vi "CVFinder.vi"() -> ()   [LabVIEW 2017]
uses:
  <vilib>/Utility/file.llb/Write Delimited Spreadsheet (string).vi
  <vilib>/Utility/file.llb/Write Delimited Spreadsheet (DBL).vi
  <instrlib>/Agilent E4980/Agilent E4980.lvlib
  <vilib>/Analysis/NI_AALPro.lvlib
panel:
  in  "Save data after run":bool=TRUE
  in  "Save NW Image to:":path=path "C:/Users/Noah/Desktop/NW_test.png" caption="Save CV Data to:"
  in  "stoploop":bool
  out "Steps":dbl
  out "Width (mm)":dbl
  out "Capacitance (pF)":dbl
  out "NW":cluster{dbl[], ext[unit][]}(graph) caption="Primary"
  out "1_C2V":cluster{dbl[], dbl[]}(graph)={[-1.0], [1.8568866883502444e+20]} caption="Primary"
  in  "Save CV Data to:":path=path "C:/Users/Noah/Desktop/CV_test.txt"
  out "CV":cluster{dbl[], dbl[]}(graph)={[-1.0], [73.385]} caption="Primary"
  in  "Manual Impedance Range (3: 100 Ohms) 2":i32(ring)=3 items=["100m", "1", "10", "100", "300", "1K", "3K", "10K", "30K", "100K"]
  in  "Relative Permittivity, er":dbl=11.68 caption="Permittivity (pF/cm)"
  in  "Signal Frequency (kHz)":dbl=1000.0
  in  "Voltage Increment (V)":dbl=0.05
  in  "Final Voltage (V)":dbl=3.0
  in  "Initial Voltage (V)":dbl=0.1
  in  "Area (cm^2)":dbl=0.005153 format="%#_6e"
  in  "Enable Auto Range (T:Enable) 2":bool=TRUE
  in  "Signal Type (0: Voltage) 2":u16(ring) items=["Voltage"]
  in  "Function (0: Cp-D) 2":u16(ring)=1 items=["Cp-D", "Cp-Q", "Cp-G", "Cp-Rp", "Cs-D", "Cs-Q", "Cs-Rs", "Lp-D", "Lp-Q", "Lp-G", "Lp-Rp", "Lp-Rdc", "Ls-D", "Ls-Q", "Ls-Rs", "Ls-Rdc", "R-X", "Z-thd", "Z-thr", "G-B", "Y-thd", "Y-thr", "Vdc-Idc"]
  in  "error in (no error)":errorcluster
  in  "VISA resource name":refnum<visa-resource-name>="USB0::0x0957::0x0909::MY46101893::INSTR"
  out "Q":dbl
  # "e0 = 0.088542 pF/cm"
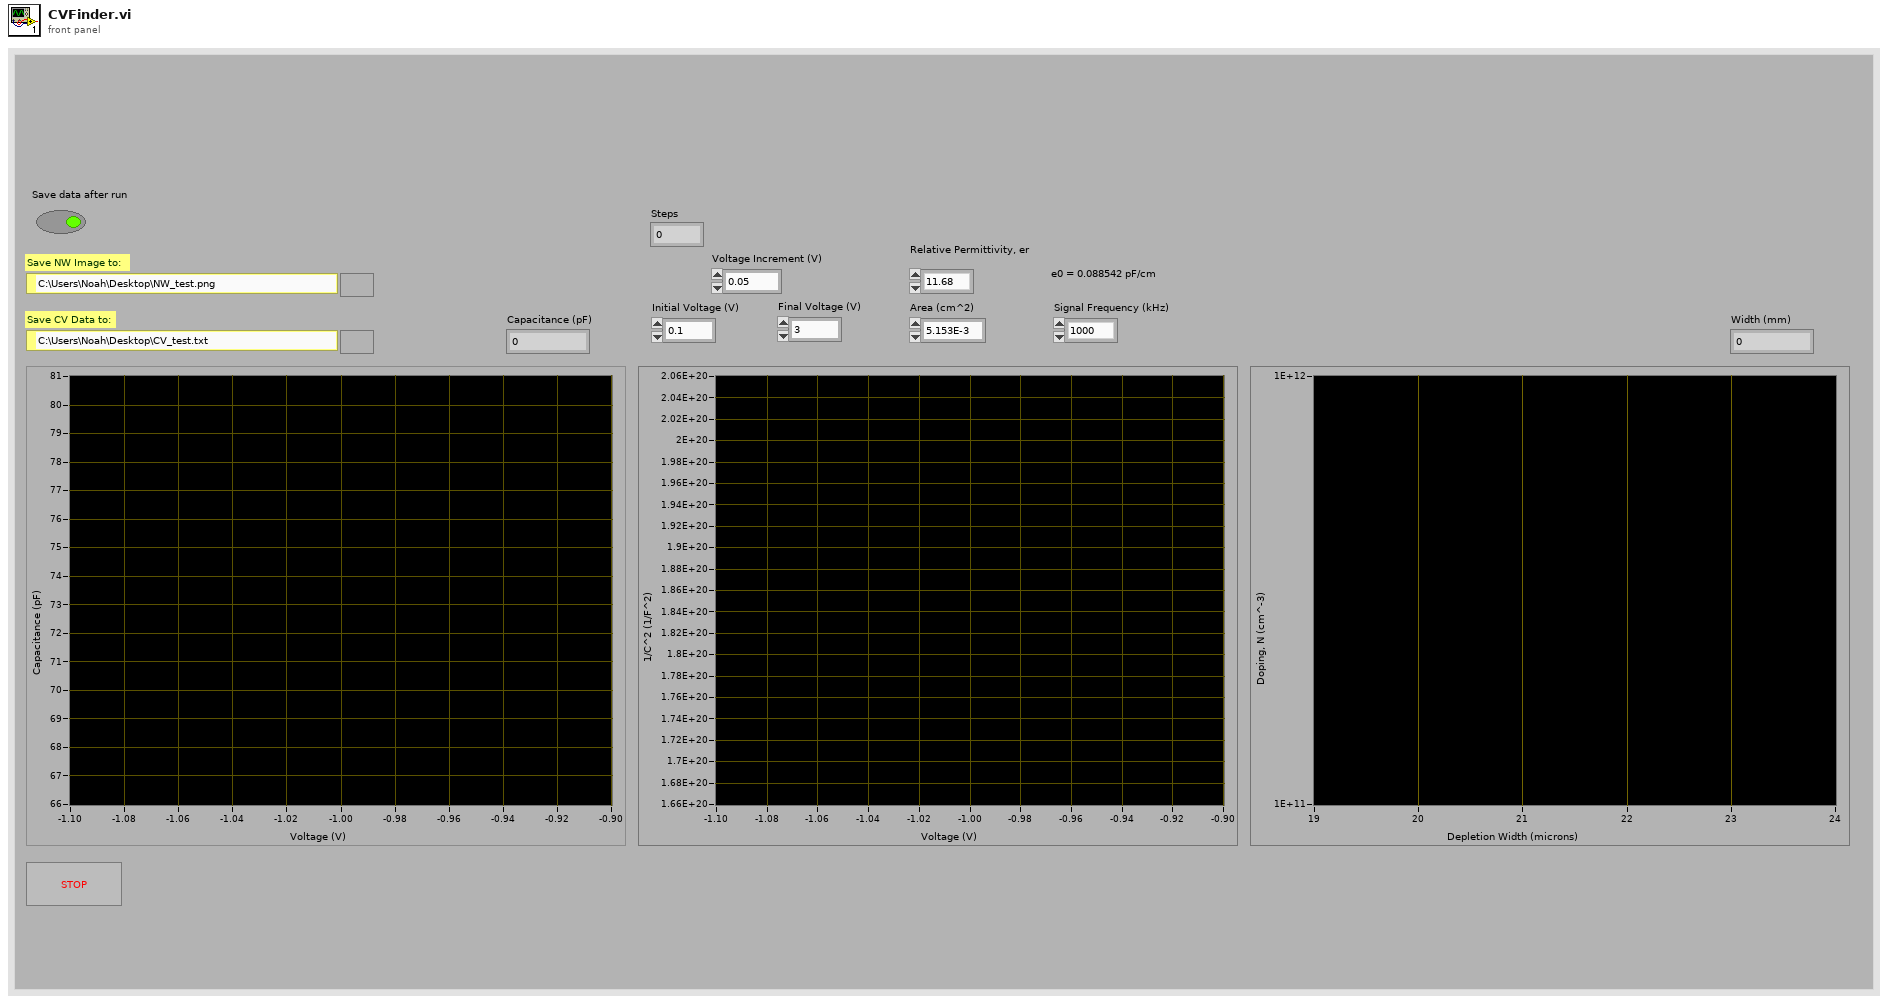
[diagram p1: front panel]
types:
  T1 = typedef "imagedata.ctl" = cluster{"image type":i32, "image depth":i32, "image":u8[], "mask":u8[], "colors":u32[], "Rectangle":cluster{"left":i16, "top":i16, "right":i16, "bottom":i16}}
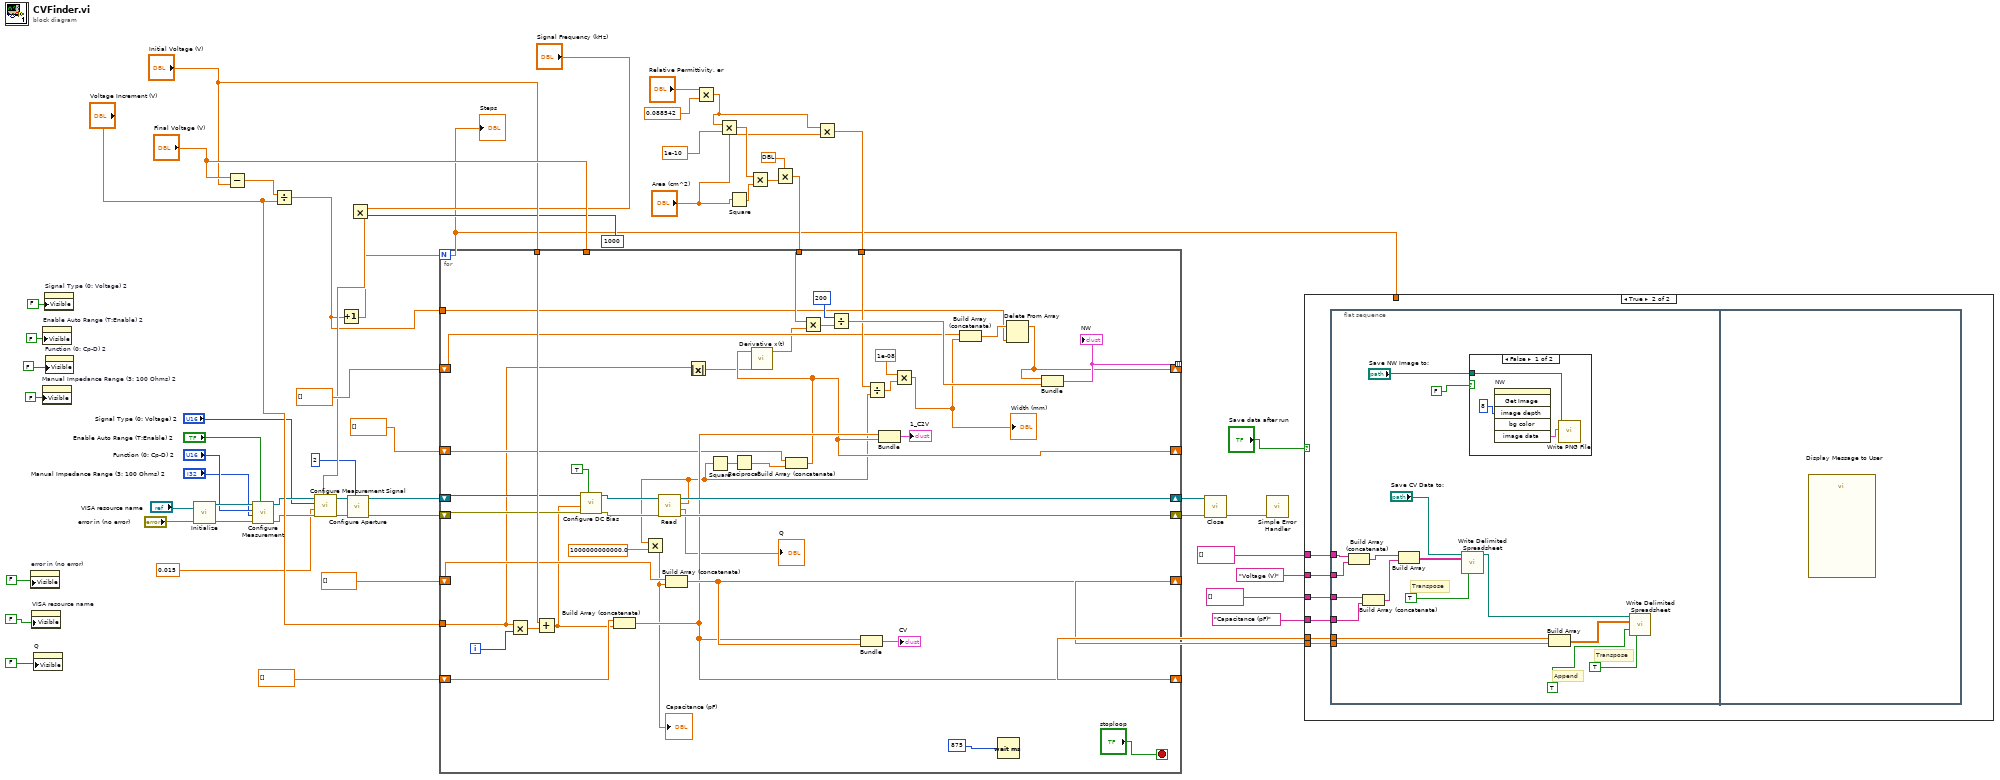
[diagram p0: block diagram]
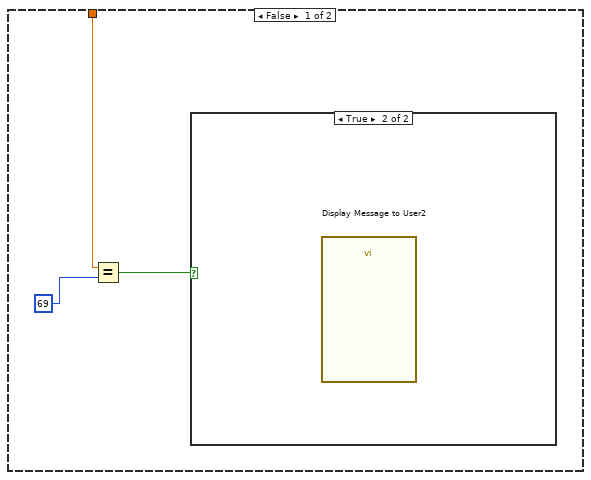
[diagram p2: hidden frame]
diagram:
  n1 = property on="error in (no error)" class="Clust (strict)"("Visible"=FALSE) -> ()  [unwired: 2 in, 2 out]
  n2 = property on="VISA resource name" class="VISAName"("Visible"=FALSE) -> ()  [unwired: 2 in, 2 out]
  n3 = property on="Q" class="DigNum (strict)"("Visible"=FALSE) -> ()  [unwired: 2 in, 2 out]
  n4 = property on="Manual Impedance Range (3: 100 Ohms) 2" class="Ring (strict)"("Visible"=FALSE) -> ()  [unwired: 2 in, 2 out]
  n5 = property on="Enable Auto Range (T:Enable) 2" class="Bool (strict)"("Visible"=FALSE) -> ()  [unwired: 2 in, 2 out]
  n6 = property on="Signal Type (0: Voltage) 2" class="Ring (strict)"("Visible"=FALSE) -> ()  [unwired: 2 in, 2 out]
  n7 = property on="Function (0: Cp-D) 2" class="Ring (strict)"("Visible"=FALSE) -> ()  [unwired: 2 in, 2 out]
  n8 = call <instrlib>:"Initialize.vi"("error in (no error)"="error in (no error)", "VISA resource name"="VISA resource name") -> ("error out"=w51:errorcluster, "VISA resource name out"=w52:refnum<visa-resource-name>)  [unwired: 8 in]
  n9 = Subtract(x="Final Voltage (V)", y="Initial Voltage (V)") -> (x-y=w56:dbl)
  n10 = call <instrlib>:"Configure Measurement.vi"("Enable Auto Range (T:Enable)"="Enable Auto Range (T:Enable) 2", "error in (no error)"=w51, "Manual Impedance Range (3: 100 Ohms)"="Manual Impedance Range (3: 100 Ohms) 2", "Function (0: Cp-D)"="Function (0: Cp-D) 2", "VISA resource name"=w52) -> ("error out"=w27:errorcluster, "VISA resource name out"=w26:refnum<visa-resource-name>)  [unwired: 5 in]
  n11 = Divide(x=w56, y="Voltage Increment (V)") -> (x/y=w14:dbl)
  n12 = Increment(x=w14) -> (x+1=w1:dbl)
  "Steps" <- w1
  n13 = Multiply(x="Signal Frequency (kHz)", y=1000) -> (x*y=w24:dbl)
  n14 = call <instrlib>:"Configure Measurement Signal.vi"("Signal Frequency (1000 Hz)"=w24, "error in (no error)"=w27, "Signal Level (1.0 V)"=0.015, "Signal Type (0: Voltage)"="Signal Type (0: Voltage) 2", "VISA resource name"=w26) -> ("error out"=w22:errorcluster, "VISA resource name out"=w21:refnum<visa-resource-name>)  [unwired: 5 in]
  n15 = call <instrlib>:"Configure Aperture.vi"("error in (no error)"=w22, "Measurement Time (1: Medium)"=2, "VISA resource name"=w21) -> ("error out"=w18:errorcluster, "VISA resource name out"=w19:refnum<visa-resource-name>)  [unwired: 7 in]
  n16 = Multiply(x="Relative Permittivity, er", y=0.088542) -> (x*y=w15:dbl)
  n17 = Multiply(x=w15, y=1e-10) -> (x*y=w35:dbl)
  n18 = Square(x="Area (cm^2)") -> (x^2=w40:dbl)
  n19 = Multiply(x=w35, y=w40) -> (x*y=w39:dbl)
  n20 = Multiply(x=ext[unit] 1.6021766208e-19, y=w39) -> (x*y=w38:ext[unit])
  n21 = Multiply(x=w15, y="Area (cm^2)") -> (x*y=w34:dbl)
  n22 = for {
    N: w1 -> [_]
    tunnel: "Voltage Increment (V)" -> [w65]
    tunnel: "Final Voltage (V)" -> [_]
    tunnel: "Initial Voltage (V)" -> [w89]
    shift-right: [w83] -> w41
    shift-left: dbl[] [] -> [w100]
    shift-right: [w88] -> w33
    shift-left: dbl[] [] -> [w82]
    tunnel: w38 -> [w94]
    tunnel: w34 -> [w86]
    shift-right: [w67] -> _
    shift-left: dbl[] [] -> [w80]
    shift-right: [w68] -> _
    shift-left: dbl[] [] -> [w71]
    tunnel: [w79] -> _ mode=indexing
    shift-right: [w98] -> w42
    shift-left: w18 -> [w77]
    shift-right: [w85] -> w43
    shift-left: w19 -> [w78]
    tunnel: w14 -> [w69]
    i -> [w58]
    stop <- "stoploop" stop-if-true
    n23 = Multiply(x=w65, y=w58) -> (x*y=w90:dbl)
    n24 = Add(x=w89, y=w90) -> (x+y=w74:dbl)
    n25 = call <instrlib>:"Configure DC Bias.vi"("DC Bias State (F:Disable)"=TRUE, "error in (no error)"=w77, "DC Bias Level (0.0 V)"=w74, "VISA resource name"=w78) -> ("error out"=w76:errorcluster, "VISA resource name out"=w75:refnum<visa-resource-name>)  [unwired: 6 in]
    n26 = Build Array (concatenate)(w100, w74) -> (w83:dbl[])
    n27 = call <instrlib>:"Read.vi"("error in (no error)"=w76, "VISA resource name"=w75) -> ("error out"=w98:errorcluster, "Secondary Parameter"=→"Q":dbl, "Primary Parameter"=w61:dbl, "VISA resource name out"=w85:refnum<visa-resource-name>)  [unwired: 6 in]
    n28 = Multiply(x=w61, y=1000000000000.0) -> (x*y=w81:dbl)
    "Capacitance (pF)" <- w81
    n29 = Build Array (concatenate)(w82, w81) -> (w88:dbl[])
    n30 = Absolute Value(x=w65) -> (abs(x)=w64:dbl)
    n31 = Square(x=w61) -> (x^2=w96:dbl)
    n32 = Reciprocal(x=w96) -> (1/x=w84:dbl)
    n33 = Build Array (concatenate)(w80, w84) -> (w67:dbl[])
    n34 = call <vilib>:"Derivative x(t).vi"("dt"=w64, "X"=w67) -> ("dX/dt"=w66:dbl[])  [unwired: 8 in, 1 out]
    n35 = Multiply(x=w94, y=w66) -> (x*y=w93:ext[unit][])
    n36 = Divide(x=200, y=w93) -> (x/y=w92:ext[unit][])
    n37 = Bundle(w83, w88) -> (→"CV":cluster{dbl[], dbl[]})  [unwired: 1 out]
    n38 = Divide(x=w86, y=w61) -> (x/y=w63:dbl)
    n39 = Bundle(w83, w67) -> (→"1_C2V":cluster{dbl[], dbl[]})  [unwired: 1 out]
    n40 = Multiply(x=1e-08, y=w63) -> (x*y=w60:dbl)
    "Width (mm)" <- w60
    n41 = Build Array (concatenate)(w71, w60) -> (w70:dbl[])
    n42 = Wait (ms)(milliseconds to wait=875) -> ()  [unwired: 1 out]
    n43 = Delete From Array(array=w70, index=w69) -> (array with subset deleted=w68:dbl[])  [unwired: 1 in, 1 out]
    n44 = Bundle(w68, w92) -> (w79:cluster{dbl[], ext[unit][]})  [unwired: 1 out]
    "NW" <- w79
  }
  n45 = call <instrlib>:"Close.vi"("error in (no error)"=w42, "VISA resource name"=w43) -> ("error out"=w44:errorcluster)  [unwired: 9 in]
  n46 = call <vilib>:"Simple Error Handler.vi"("error in (no error)"=w44) -> ()  [unwired: 4 in, 5 out]
  n47 = case shown="True" "Save data after run" {
    tunnel: w41 -> [_ w109]
    tunnel: w33 -> [_ w108]
    tunnel: string[] [] -> [_ w107]
    tunnel: string[] [] -> [_ w106]
    tunnel: "Voltage (V)" -> [_ w105]
    tunnel: "Capacitance (pF)" -> [_ w104]
    tunnel: w1 -> [w101 _]
    frame False {
      n48 = Equal?(x=w101, y=69) -> (x = y?=w102:bool)
      n49 = case shown="True" w102 {
        frame False {
        }
        frame True {
          n50 = call "Display Message to User2"() -> ()  [unwired: 10 in, 2 out]
        }
      }
    }
    frame True {
      n51 = flat-sequence {
        tunnel: w109 -> [w126]
        tunnel: w108 -> [w125]
        tunnel: w107 -> [w124]
        tunnel: w106 -> [w123]
        tunnel: w105 -> [w122]
        tunnel: w104 -> [w121]
        frame #0 {
          # "Append"
          # "Transpose"
          # "Transpose"
          n52 = Build Array (concatenate)(w123, w122) -> (w113:string[])
          n53 = Build Array (concatenate)(w124, w121) -> (w114:string[])
          n54 = Build Array(w113, w114) -> (w115:string[][])
          n55 = call-poly <vilib>:"Write Delimited Spreadsheet.vi"("file path (dialog if empty)"="Save CV Data to:", "2D data"=w115, "transpose? (no:F)"=TRUE) -> ("new file path (Not A Path if cancelled)"=w117:path)  [unwired: 11 in, 1 out]
          n56 = case shown="False" FALSE {
            tunnel: "Save NW Image to:" -> [w129 _]
            frame False {
              n57 = invoke on="NW" class="XYGraph (strict)" method="Get Image"("image depth"=8) -> ("image data"=w127:T1)  [unwired: 5 in, 5 out]
              n58 = call <vilib>:"Write PNG File.vi"("image data"=w127, "path to PNG file"=w129) -> ()  [unwired: 8 in, 2 out]
            }
            frame True {
            }
          }
          n59 = Build Array(w126, w125) -> (w120:dbl[][])
          n60 = call-poly <vilib>:"Write Delimited Spreadsheet.vi"("file path (dialog if empty)"=w117, "2D data"=w120, "append to file? (new file:F)"=TRUE, "transpose? (no:F)"=TRUE) -> ()  [unwired: 10 in, 2 out]
        }
        frame #1 {
          n61 = call "Display Message to User"() -> ()  [unwired: 10 in, 2 out]
        }
      }
    }
  }
